vi "3-6.vi"() -> ()   [LabVIEW 2014]
panel:
  in  "Boolean 2":bool
  in  "Boolean":bool
  out "Numeric 2":dbl
  out "Numeric":dbl
  in  "Fahrenheit":dbl
  in  "Celsius":dbl
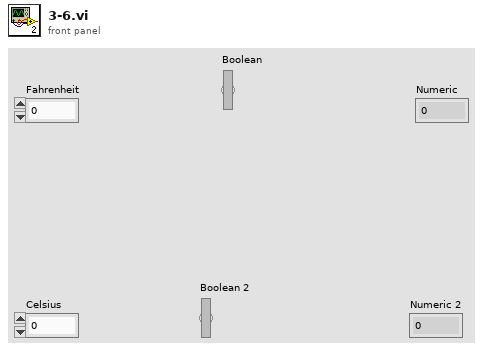
[diagram p1: front panel]
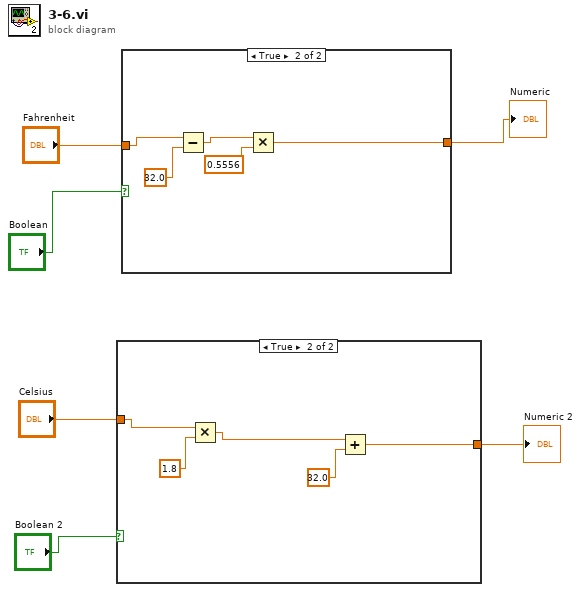
[diagram p0: block diagram]
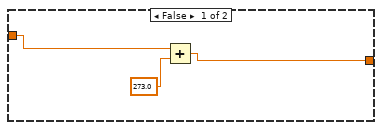
[diagram p2: hidden frame]
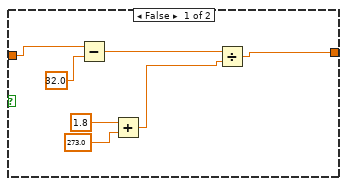
[diagram p3: hidden frame]
diagram:
  n1 = case shown="True" "Boolean 2" {
    tunnel: "Celsius" -> [w9 w13]
    tunnel: [w7 w10] -> w3
    frame False {
      n2 = Add(x=w9, y=273.0) -> (x+y=w7:dbl)
    }
    frame True {
      n3 = Multiply(x=w13, y=1.8) -> (x*y=w12:dbl)
      n4 = Add(x=w12, y=32.0) -> (x+y=w10:dbl)
    }
  }
  "Numeric 2" <- w3
  n5 = case shown="True" "Boolean" {
    tunnel: "Fahrenheit" -> [w21 w26]
    tunnel: [w15 w22] -> w5
    frame False {
      n6 = Subtract(x=w21, y=32.0) -> (x-y=w17:dbl)
      n7 = Add(x=1.8, y=273.0) -> (x+y=w16:dbl)
      n8 = Divide(x=w17, y=w16) -> (x/y=w15:dbl)
    }
    frame True {
      n9 = Subtract(x=w26, y=32.0) -> (x-y=w24:dbl)
      n10 = Multiply(x=w24, y=0.5556) -> (x*y=w22:dbl)
    }
  }
  "Numeric" <- w5
